vi "Example.vi"() -> ()   [LabVIEW 2018]
uses:
  Data Def/FATEK-Request Message Format.ctl
  Data Def/FATEK-Command Code.ctl
  Data Def/FATEK-Write to multiple consecutive registers.ctl
  Data Def/FATEK-Device Code.ctl
  Data Def/FATEK-Read multiple data of consecutive registers.ctl
  Data Def/FATEK-Read Response Message.ctl
panel:
  out "Numeric":i32
  in  "Tab Control":enum32{"Read", "Write"}(tab)
  in  "Read multiple data of consecutive registers":T1={"Number N"=50, "Device Code"=enum."D", "Start Position"=0}
  out "Data":bool[][](array[boolean])
  in  "Write to multiple consecutive registers":T2
  out "Read Response Message":T4={"Slave Station No"="01", "Command Code"=72, "Error Code"=0, "Response Data"=[]} {"Command Code" items=["Read multiple data of consecutive registers"=70, "Write to multiple consecutive registers"=71]}
  out "Time":u32
  out "Bytes To Read":i32
  out "Request Message":string
  out "error out":errorcluster
  out "Response Data":string
  in  "Stop":bool
  in  "Request Message Format":T6={"Slave Station No"="01", "Command Code"=70, "Control Code"=variant} {"Command Code" items=["Read multiple data of consecutive registers"=70, "Write to multiple consecutive registers"=71]}
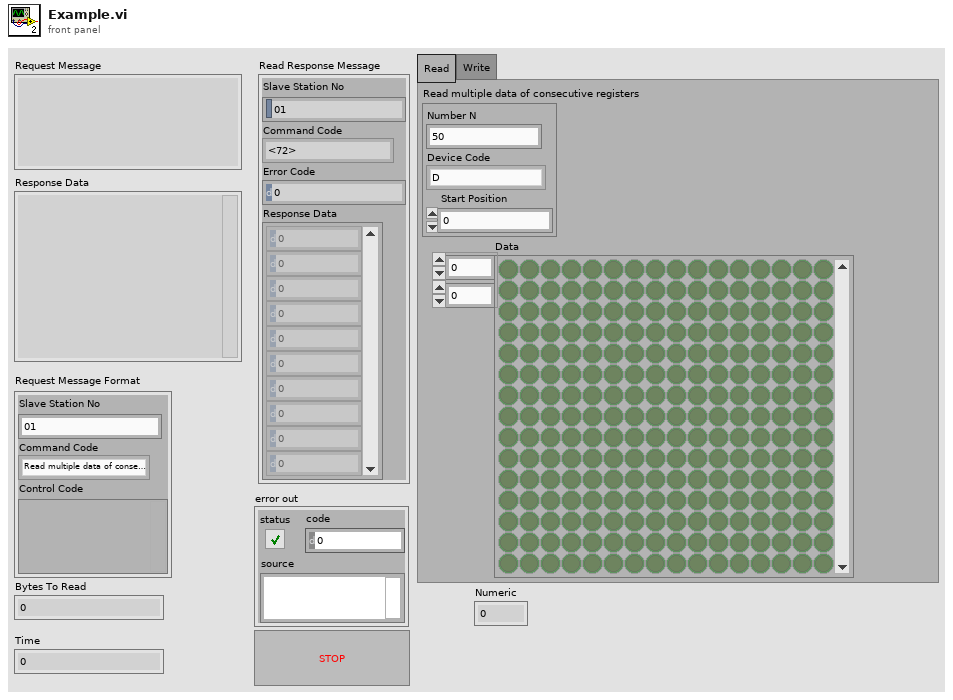
[diagram p1: front panel]
types:
  T1 = typedef "FATEK-Read multiple data of consecutive registers.ctl" = cluster{"Number N":u8, "Device Code":enum16{"X", "Y", "M", "R", "D"}, "Start Position":u16}
  T2 = typedef "FATEK-Write to multiple consecutive registers.ctl" = cluster{"Number N":u8, "Device Code":T3, "Position":u16, "Value":i16[]}
  T3 = typedef "FATEK-Device Code.ctl" = enum16{"X", "Y", "M", "R", "D"}
  T4 = typedef "FATEK-Read Response Message.ctl" = cluster{"Slave Station No":string, "Command Code":T5, "Error Code":u8, "Response Data":i16[]}
  T5 = typedef "FATEK-Command Code.ctl" = u16
  T6 = typedef "FATEK-Request Message Format.ctl" = cluster{"Slave Station No":string, "Command Code":T5, "Control Code":variant}
  T7 = enum16{"Standard", "Buffered", "CRLF", "Immediate"}
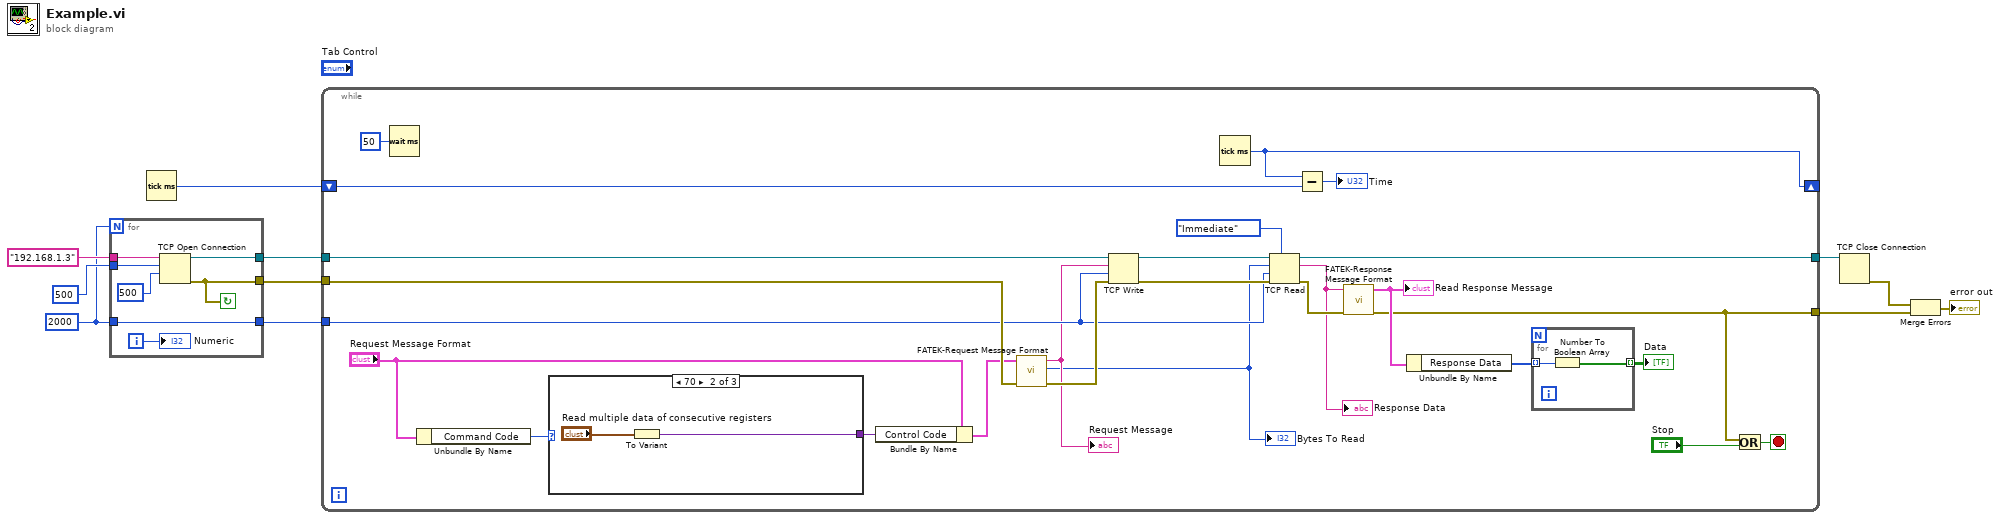
[diagram p0: block diagram]
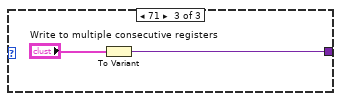
[diagram p3: hidden frame]
diagram:
  w1 = 2000 ("timeout ms (60000)")
  n1 = for {
    N: w1 -> [_]
    tunnel: "192.168.1.3" ("address") -> [w18]
    tunnel: [w17] -> w10
    tunnel: [w13] -> w5
    tunnel: u16 500 ("remote port or service name") -> [w16]
    tunnel: w1 -> [w15]
    tunnel: [w15] -> w2
    i -> [w12]
    stop <- w13 continue-if-true
    n2 = TCP Open Connection(address=w18, remote port or service name=w16, timeout ms (60000)=500) -> (connection ID=w17:refnum<k5>, error out=w13:errorcluster)  [unwired: 2 in]
    "Numeric" <- w12
  }
  n3 = Tick Count (ms)() -> (millisecond timer value=w4:u32)
  n4 = while {
    tunnel: w10 -> [w44]
    tunnel: w5 -> [w43]
    tunnel: w2 -> [w38]
    tunnel: [w21] -> w7
    tunnel: [w39] -> w9
    shift-right: [w33] -> _
    shift-left: w4 -> [w34]
    stop <- w19 stop-if-true
    n5 = Wait (ms)(milliseconds to wait=u32 50) -> ()  [unwired: 1 out]
    n6 = Unbundle By Name("Request Message Format") -> ("Command Code"=w30:T5)
    n7 = case shown="70" w30 {
      tunnel: [_ w48 w50] -> w28
      frame Default {
      }
      frame 70 {
        n8 = To Variant(anything="Read multiple data of consecutive registers") -> (Variant=w48:variant)
      }
      frame 71 {
        n9 = To Variant(anything="Write to multiple consecutive registers") -> (Variant=w50:variant)
      }
    }
    n10 = Bundle By Name(cluster="Request Message Format", "Control Code"=w28) -> (w27:T6)
    n11 = call "FATEK-Request Message Format.vi"("error in"=w43, "Request Message Format"=w27) -> ("error out"=w42:errorcluster, "Bytes To Read"=w35:i32, "Request Message"=w37:string)  [unwired: 7 in]
    "Request Message" <- w37
    "Bytes To Read" <- w35
    n12 = TCP Write(connection ID=w44, data in=w37, error in (no error)=w42, 9:w38) -> (connection ID out=w40:refnum<k5>, error out=w41:errorcluster)  [unwired: 1 out]
    n13 = Tick Count (ms)() -> (millisecond timer value=w33:u32)
    n14 = TCP Read(connection ID=w40, bytes to read=w35, error in (no error)=w41, 7:T7."Immediate" ("mode (standard)"), 9:w38) -> (connection ID out=w39:refnum<k5>, data out=w25:string, error out=w26:errorcluster)
    "Response Data" <- w25
    n15 = Subtract(x=w33, y=w34) -> (x-y=→"Time":u32)
    n16 = call "FATEK-Response Message Format.vi"("error in"=w26, "Response Data"=w25) -> ("error out"=w21:errorcluster, "Read Response Message"=w24:T4)  [unwired: 8 in]
    "Read Response Message" <- w24
    n17 = Unbundle By Name(w24) -> ("Response Data"=w23:i16[])
    n18 = for {
      tunnel: w23 -> [w46] mode=indexing
      tunnel: [w45] -> w22 mode=indexing
      n19 = Number To Boolean Array(number=w46) -> (Boolean array=w45:bool[])
    }
    "Data" <- w22
    n20 = Or(x=w21, y="Stop") -> (x .or. y?=w19:bool)
  }
  n21 = TCP Close Connection(connection ID=w9) -> (error out=w8:errorcluster)  [unwired: 2 in, 1 out]
  n22 = Merge Errors(w8, w7) -> (→"error out":errorcluster)
